vi "GET_Snapshot_item_by_id.vi"(9 "Item":string, 10 "SnapID":string, 11 "API Key":string="cheia04042025tema2restfulapi") -> (2 "Diagnose snapshot":string, 3 "headers":string)   [LabVIEW 2024]
uses:
  <vilib>/httpClient/LabVIEWHTTPClient.lvlib
panel:
  out "error out get":errorcluster
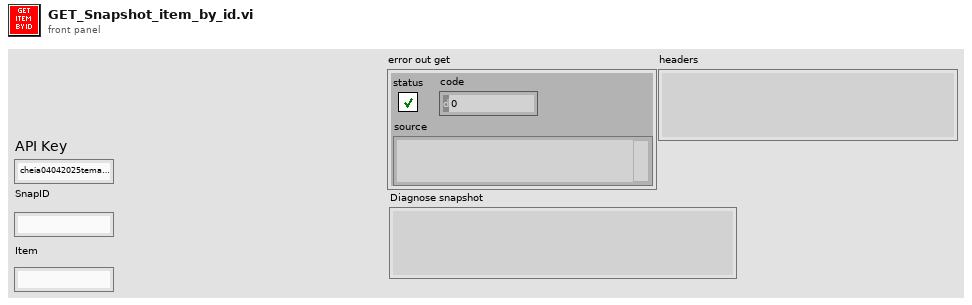
[diagram p1: front panel]
types:
  T1 = typedef "LabVIEWHTTPClient.lvlib/ClientHandle.ctl" = refnum<k1>
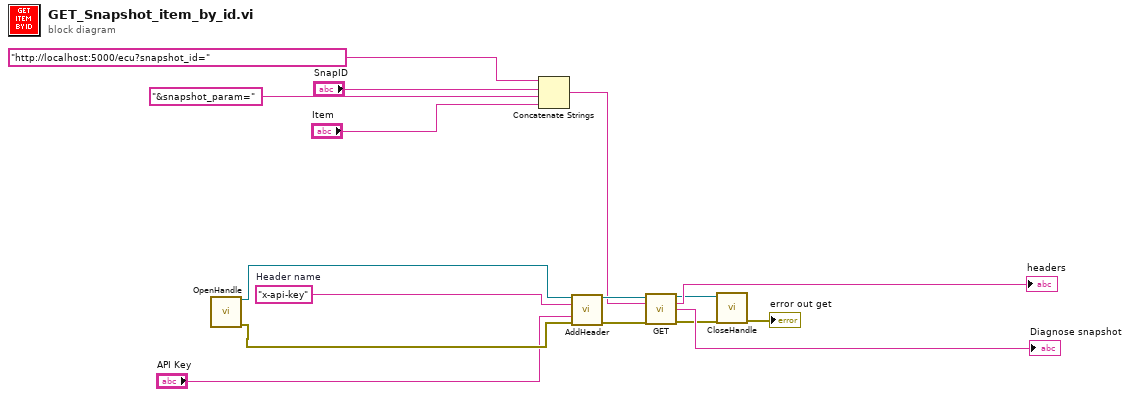
[diagram p0: block diagram]
diagram:
  w7 = "x-api-key"  # Header name
  n1 = call <vilib>:"OpenHandle.vi"() -> ("client handle out"=w8:T1, "error out"=w9:errorcluster)  [unwired: 14 in]
  n2 = Concatenate Strings("http://localhost:5000/ecu?snapshot_id=" ("url"), "SnapID", "&snapshot_param=", "Item") -> (w5:string)
  n3 = call <vilib>:"AddHeader.vi"("client handle"=w8, "header"=w7, "value"="API Key", "error in (no error)"=w9) -> ("client handle out"=w11:T1, "error out"=w10:errorcluster)  [unwired: 10 in]
  n4 = call <vilib>:"GET.vi"("client handle"=w11, "url"=w5, "error in (no error)"=w10) -> ("client handle out"=w13:T1, "headers"=→"headers":string, "body"=→"Diagnose snapshot":string, "error out"=w12:errorcluster)  [unwired: 9 in]
  n5 = call <vilib>:"CloseHandle.vi"("client handle"=w13, "error in (no error)"=w12) -> ("error out"=→"error out get":errorcluster)  [unwired: 13 in]
